vi "Configure Websockets Connection.vi"(5 "WSConnection in":refnum<class "WebsocketsConnection.lvclass">, 6 "timeout (5000 ms)":i32=5000, 8 "error in (no error)":errorcluster, 9 "path":string, 10 "remote port (80)":u16=80, 11 "address (localhost)":string="localhost") -> (0 "error out":errorcluster, 3 "WSConnection":refnum<class "WebsocketsConnection.lvclass">)   [LabVIEW 2013, in "MQTT_Websockets.lvlib" / "WebsocketsConnection.lvclass"]
uses:
  WebsocketsConnection.lvclass
  <vilib>/MediaMongrels Ltd/WebSockets/WebSockets/WebSocket/Headers.ctl
  <vilib>/MediaMongrels Ltd/WebSockets/WebSockets/WebSocket/WebSocket.lvclass
  WebsocketsConnection.lvclass/WebsocketsConnection.ctl
  <vilib>/LabVIEW Open Source Project/MQTT Connection/MQTT_Connection/Connection/Connection.lvclass/Connection.ctl
  <vilib>/LabVIEW Open Source Project/MQTT Connection/MQTT_Connection/Connection/Connection.lvclass
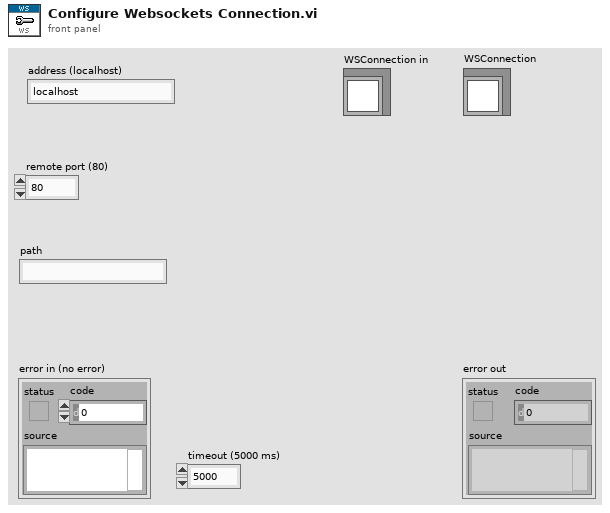
[diagram p1: front panel]
types:
  T1 = typedef "WebSockets.lvlib/WebSocket.lvclass/Headers.ctl" = cluster{"Name":string, "Value":string}
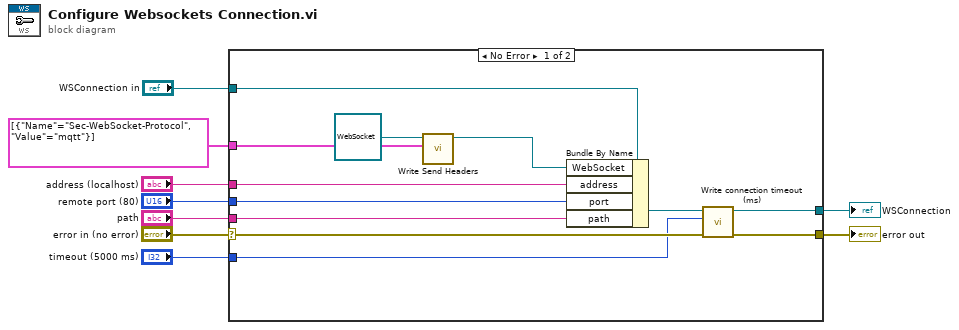
[diagram p0: block diagram]
diagram:
  n1 = case shown="No Error" "error in (no error)" {
    selector: "error in (no error)" -> [w18 w23]
    tunnel: [w15 w23] -> w8
    tunnel: [w16 w22] -> w4
    tunnel: "address (localhost)" -> [w21 _]
    tunnel: "remote port (80)" -> [w20 _]
    tunnel: "timeout (5000 ms)" -> [w17 _]
    tunnel: "path" -> [w14 _]
    tunnel: T1[] [{"Name"="Sec-WebSocket-Protocol", "Value"="mqtt"}] ("additional send headers (none)") -> [w13 _]
    tunnel: "WSConnection in" -> [w10 w22]
    frame No Error {
      n2 = call <vilib>:"Write Send Headers.vi"("additional send headers (none)"=w13, "WebSockets in"=refnum<class "WebSocket.lvclass"> refnum) -> ("WebSockets out"=w12:refnum<class "WebSocket.lvclass">)  [unwired: 8 in, 1 out]
      n3 = Bundle By Name(cluster=w10, "WebSocket"=w12, "address"=w21, "port"=w20, "path"=w14) -> (w19:refnum<class "WebsocketsConnection.lvclass">)
      n4 = call <vilib>:"Write connection timeout (ms).vi"("error in (no error)"=w18, "connection timeout (ms)"=w17, "Connection in"=w19) -> ("error out"=w15:errorcluster, "Connection out"=w16:refnum<class "WebsocketsConnection.lvclass">)  [unwired: 7 in]
    }
    frame Error {
    }
  }
  "error out" <- w8
  "WSConnection" <- w4
